vi "PalmSense Data Mesuarement.vi"(8 "error in (no error)":errorcluster, 9 "Message Data":variant, 11 "Hardware Resources in":T1) -> (0 "error out":errorcluster, 2 "Message Data Out":variant, 3 "Hardware Resources out":T1)   [LabVIEW 2020, in "PalmSens.lvlib"]
doc: "Generates sample waveforms according to the signal type in the HW Config input."
uses:
  PalmSens.lvlib
  PalmSense Hardware Configuration.ctl
  <instrlib>/PalmSens SDK for LabVIEW 5.10/PalmSens/PalmSens.lvclass
  support/Message Queue/Message Cluster.ctl
  support/HW Message Cluster.ctl
  support/PCT FGV CMD.ctl
  support/Message Queue/Enqueue Message (Single).vi
  C:/Program Files (x86)/National Instruments/LabVIEW 2020/instr.lib/PalmSens SDK for LabVIEW 5.10/PalmSens/Libraries/PalmSens.Core.dll
  support/Message Queue/Message Queue.lvlib
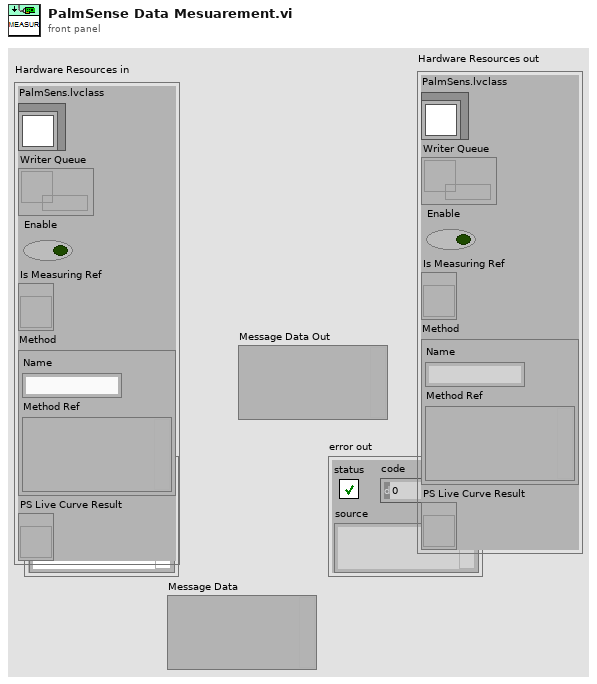
[diagram p1: front panel]
types:
  T1 = typedef "PalmSens.lvlib/PalmSense Hardware Configuration.ctl" = cluster{"PalmSens.lvclass":refnum<class "PalmSens.lvclass">, "Writer Queue":refnum<queue>, "Enable":bool, "Is Measuring Ref":refnum<vi>, "Method":cluster{"Name":string, "Method Ref":variant}, "PS Live Curve Result":refnum<vi>}
  T2 = typedef "PCT FGV CMD.ctl" = enum16{"INIT", "GET", "SET"}
  T3 = typedef "Message Queue.lvlib/HW Message Cluster.ctl" = cluster{"Writer Queue":refnum<queue>, "Writer Data":T4}
  T4 = typedef "Message Queue.lvlib/Message Cluster.ctl" = cluster{"Message":string, "Message Data":variant}
  T5 = typedef "MeasurementResults.ctl" = T6[]
  T6 = typedef "LiveCurveResult.ctl" = cluster{"X Label":string, "Y Label":string, "Name":string, "Index":i16, "Curve Values":cluster{"Values":cluster{"X Value":dbl, "Y Value":dbl}[], "Index":i16}}
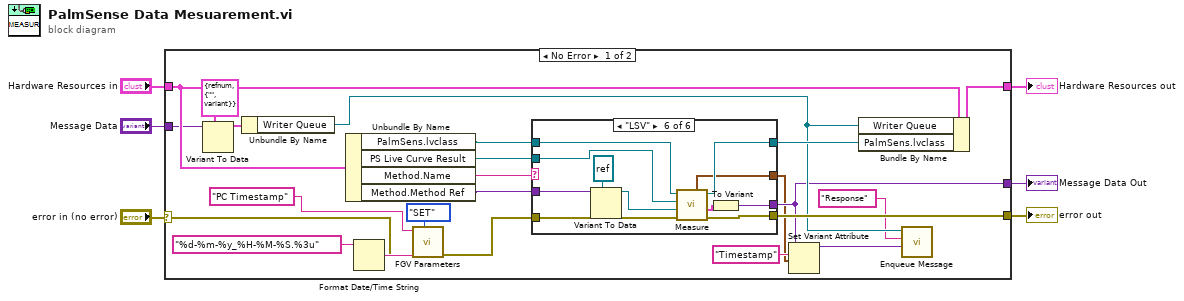
[diagram p0: block diagram]
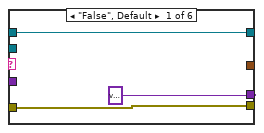
[diagram p2: hidden frame]
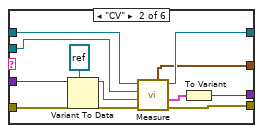
[diagram p3: hidden frame]
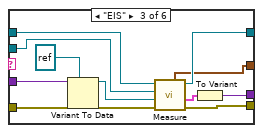
[diagram p4: hidden frame]
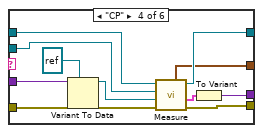
[diagram p5: hidden frame]
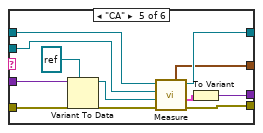
[diagram p6: hidden frame]
diagram:
  n1 = case shown="No Error" "error in (no error)" {
    selector: "error in (no error)" -> [w8 w89]
    tunnel: [w27 w89] -> w5
    tunnel: [w18 _] -> w4
    tunnel: "Hardware Resources in" -> [w29 w88]
    tunnel: [w28 w88] -> w2
    tunnel: "Message Data" -> [w24 _]
    frame No Error {
      n2 = Variant To Data(type=T3 {"Writer Queue"=refnum, "Writer Data"={"Message"="", "Message Data"=variant}}, Variant=w24) -> (data=w25:T3)  [unwired: 1 in, 1 out]
      n3 = Unbundle By Name(w25) -> ("Writer Queue"=w20:refnum<queue>)
      n4 = Unbundle By Name(w29) -> ("PalmSens.lvclass"=w22:refnum<class "PalmSens.lvclass">, "PS Live Curve Result"=w17:refnum<vi>, "Method.Name"=w13:string, "Method.Method Ref"=w23:variant)
      n5 = Format Date/Time String(time format string (%c)="%d-%m-%y_%H-%M-%S.%3u") -> (date/time string=w9:string)  [unwired: 2 in]
      n6 = call "FGV Parameters.vi"("CMD"=PCT_FGV_CMD."SET", "error in (no error)"=w8, "input"=w9, "Key"="PC Timestamp") -> ("error out"=w7:errorcluster)  [unwired: 5 in, 2 out]
      n7 = case shown="\"LSV\"" w13 {
        tunnel: [variant ("Variant") w34 w45 w56 w67 w78] -> w18
        tunnel: [w30 w36 w48 w59 w70 w80] -> w21
        tunnel: w7 -> [w31 w39 w51 w62 w73 w83]
        tunnel: [w31 w38 w50 w61 w72 w82] -> w27
        tunnel: w23 -> [_ w43 w54 w65 w76 w87]
        tunnel: w22 -> [w30 w40 w52 w63 w74 w84]
        tunnel: w17 -> [_ w35 w46 w57 w68 w79]
        tunnel: [_ w33 w44 w55 w66 w77] -> w14
        frame "False", Default {
        }
        frame "CV" {
          n8 = Variant To Data(type=refnum<k24> refnum ("CV reference"), Variant=w43) -> (data=w41:refnum<k24>)  [unwired: 1 in, 1 out]
          n9 = call-dynamic "Measure.vi"("error in (no error)"=w39, "Method .NET Refnum"=w41, "Live Curve Result Refnum"=w35, "PalmSens in"=w40) -> ("error out"=w38:errorcluster, "Results"=w37:T5, "PalmSens out"=w36:refnum<class "PalmSens.lvclass">, "TimeStamp"=w33:timestamp)  [unwired: 4 in]
          n10 = To Variant(anything=w37) -> (Variant=w34:variant)
        }
        frame "EIS" {
          n11 = Variant To Data(type=refnum<k24> refnum ("EIS"), Variant=w54) -> (data=w53:refnum<k24>)  [unwired: 1 in, 1 out]
          n12 = call-dynamic "Measure.vi"("error in (no error)"=w51, "Method .NET Refnum"=w53, "Live Curve Result Refnum"=w46, "PalmSens in"=w52) -> ("error out"=w50:errorcluster, "Results"=w49:T5, "PalmSens out"=w48:refnum<class "PalmSens.lvclass">, "TimeStamp"=w44:timestamp)  [unwired: 4 in]
          n13 = To Variant(anything=w49) -> (Variant=w45:variant)
        }
        frame "CP" {
          n14 = Variant To Data(type=refnum<k24> refnum ("reference out"), Variant=w65) -> (data=w64:refnum<k24>)  [unwired: 1 in, 1 out]
          n15 = call-dynamic "Measure.vi"("error in (no error)"=w62, "Method .NET Refnum"=w64, "Live Curve Result Refnum"=w57, "PalmSens in"=w63) -> ("error out"=w61:errorcluster, "Results"=w60:T5, "PalmSens out"=w59:refnum<class "PalmSens.lvclass">, "TimeStamp"=w55:timestamp)  [unwired: 4 in]
          n16 = To Variant(anything=w60) -> (Variant=w56:variant)
        }
        frame "CA" {
          n17 = Variant To Data(type=refnum<k24> refnum ("reference out"), Variant=w76) -> (data=w75:refnum<k24>)  [unwired: 1 in, 1 out]
          n18 = call-dynamic "Measure.vi"("error in (no error)"=w73, "Method .NET Refnum"=w75, "Live Curve Result Refnum"=w68, "PalmSens in"=w74) -> ("error out"=w72:errorcluster, "Results"=w71:T5, "PalmSens out"=w70:refnum<class "PalmSens.lvclass">, "TimeStamp"=w66:timestamp)  [unwired: 4 in]
          n19 = To Variant(anything=w71) -> (Variant=w67:variant)
        }
        frame "LSV" {
          n20 = Variant To Data(type=refnum<k24> refnum ("LSV reference"), Variant=w87) -> (data=w85:refnum<k24>)  [unwired: 1 in, 1 out]
          n21 = call-dynamic "Measure.vi"("error in (no error)"=w83, "Method .NET Refnum"=w85, "Live Curve Result Refnum"=w79, "PalmSens in"=w84) -> ("error out"=w82:errorcluster, "Results"=w81:T5, "PalmSens out"=w80:refnum<class "PalmSens.lvclass">, "TimeStamp"=w77:timestamp)  [unwired: 4 in]
          n22 = To Variant(anything=w81) -> (Variant=w78:variant)
        }
      }
      n23 = Set Variant Attribute(Variant=w18, name="Timestamp", value=w14) -> (Variant out=w16:variant)  [unwired: 1 in, 2 out]
      n24 = Bundle By Name(cluster=w29, "Writer Queue"=w20, "PalmSens.lvclass"=w21) -> (w28:T1)
      n25 = call-poly "Enqueue Message.vi"("Message Data"=w16, "Message"="Response", "Message Queue"=w20) -> ()  [unwired: 7 in, 2 out]
    }
    frame Error {
    }
  }
  "error out" <- w5
  "Message Data Out" <- w4
  "Hardware Resources out" <- w2
